vi "LatestImages.vi"(9 "VersionInput":string, 10 "ImageInput":string) -> (2 "Update":bool)   [LabVIEW 2017]
panel:
  in  "ImageName 2":string[](array[string])
  # "0 - CMS-9068\n1 - CMS-9065\n2 - CMS-9024\n3 - CMS-9036\n4 - MMS-9068\n5 - MMS-9065\n6 - EMSA-9068"
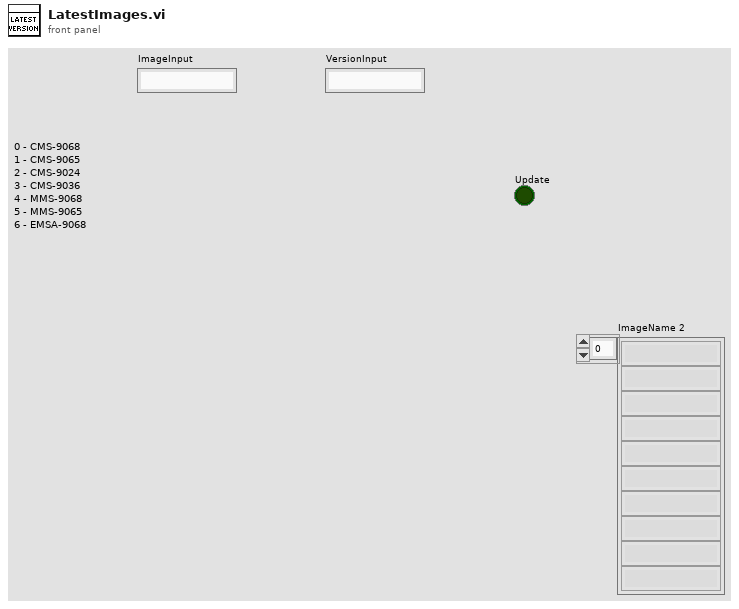
[diagram p1: front panel]
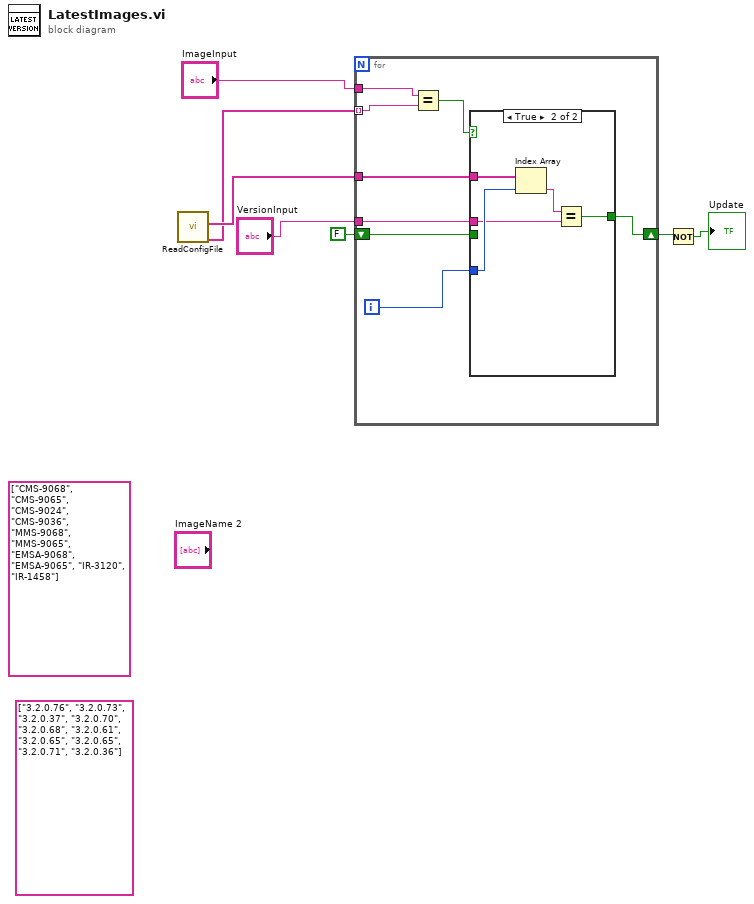
[diagram p0: block diagram]
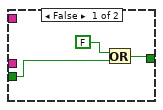
[diagram p2: hidden frame]
diagram:
  (unwired) string[] ["3.2.0.76", "3.2.0.73", "3.2.0.37", "3.2.0.70", "3.2.0.68", "3.2.0.61", "3.2.0.65", "3.2.0.65", "3.2.0.71", "3.2.0.36"] ("ImageVersion")
  (unwired) string[] ["CMS-9068", "CMS-9065", "CMS-9024", "CMS-9036", "MMS-9068", "MMS-9065", "EMSA-9068", "EMSA-9065", "IR-3120", "IR-1458"] ("ImageName")
  n1 = call "ReadConfigFile.vi"() -> ("Image Type"=w1:string[], "Versions"=w2:string[])  [unwired: 8 in, 2 out]
  n2 = for {
    tunnel: w1 -> [w15] mode=indexing
    tunnel: "ImageInput" -> [w14]
    tunnel: w2 -> [w12]
    tunnel: "VersionInput" -> [w10]
    shift-right: [w9] -> w4
    shift-left: FALSE -> [w8]
    i -> [w11]
    n3 = Equal?(x=w14, y=w15) -> (x = y?=w13:bool)
    n4 = case shown="True" w13 {
      tunnel: w12 -> [_ w23]
      tunnel: w11 -> [_ w22]
      tunnel: w10 -> [_ w20]
      tunnel: [w18 w19] -> w9
      tunnel: w8 -> [w17 _]
      frame False {
        n5 = Or(x=FALSE, y=w17) -> (x .or. y?=w18:bool)
      }
      frame True {
        n6 = Index Array(array=w23, index=w22) -> (element=w21:string)
        n7 = Equal?(x=w21, y=w20) -> (x = y?=w19:bool)
      }
    }
  }
  n8 = Not(x=w4) -> (.not. x?=→"Update":bool)
